vi "Get VI Reference.vi"(8 "error in (no error)":errorcluster, 11 "SMO UI":refnum<class "SMO.UI.lvclass">) -> (0 "error out":errorcluster, 2 "VI Reference":refnum<vi>, 3 "SMO UI out":refnum<class "SMO.UI.lvclass">)   [LabVIEW 2019, in "SMO.UI.lvclass"]
doc: "JKI State Machine Objects (SMO) 1.3.0.56\nJKI - JKI\nCopyright (c) 2017, JKI"
uses:
  SMO.UI.lvclass
  C:/Users/Patrick/Documents/GitHub/Test (LV2019)/lv-venv/lv.lib/vi.lib/JKI/JKI SMO/SMO/SMO.lvclass
  SMO/SMO.lvclass
panel:
  # "For instructions on how to use the JKI State Machine Objects, examples and video tutorials, visit:\nhttp://jki.net/state-machine-objects/\n\nJKI State Machine Objects™\nhttp://jki.net/state-machine-objects/\nCopyright (C) 2005-2015, JKI <info@jki.net>\nALL RIGHTS RESERVED"
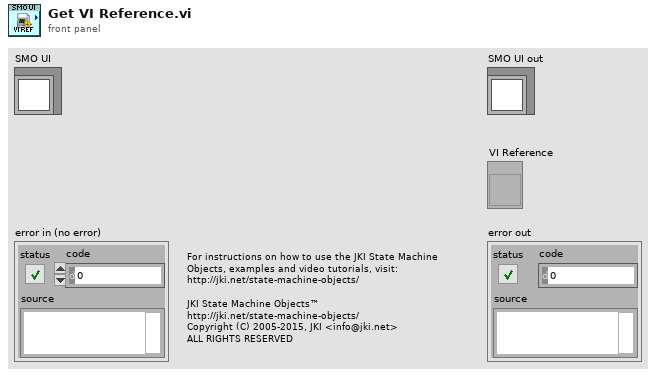
[diagram p1: front panel]
types:
  T1 = typedef "SMO.lvclass/RegisteredProcessData--Cluster.ctl" = cluster{"Name":string, "Static VI Ref":refnum<vi>, "Running":bool, "NotifierRef":u32}
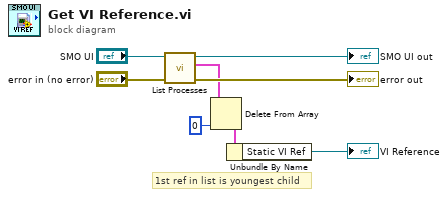
[diagram p0: block diagram]
diagram:
  # "1st ref in list is youngest child"
  n1 = call "List Processes.vi"("error in (no error)"="error in (no error)", "SMO"="SMO UI") -> ("error out"=→"error out":errorcluster, "Registered Processes"=w4:T1[], "SMO out"=→"SMO UI out":refnum<class "SMO.UI.lvclass">)  [unwired: 7 in]
  n2 = Delete From Array(array=w4, index=0) -> (deleted portion=w5:T1)  [unwired: 1 in, 1 out]
  n3 = Unbundle By Name(w5) -> ("Static VI Ref"=→"VI Reference":refnum<vi>)
